vi "Create.vi"(6 "RH?":bool, 8 "Error In":errorcluster) -> (0 "error out":errorcluster)   [LabVIEW 2017]
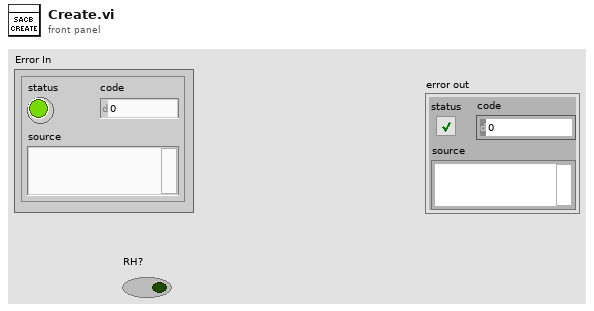
[diagram p1: front panel]
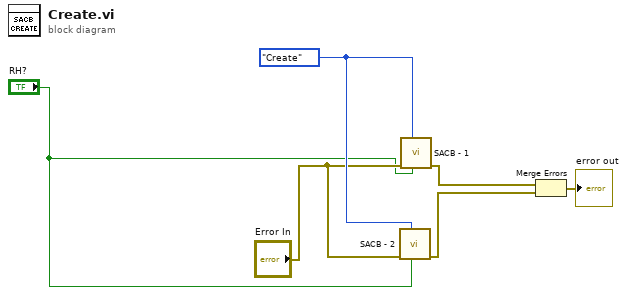
[diagram p0: block diagram]
diagram:
  w6 = enum16{"Create", "Read", "Close"}."Create" ("Command")
  n1 = call "SACB - 2.vi"("RH?"="RH?", "Command"=w6, "Error In"="Error In") -> ("Error Out"=w4:errorcluster)  [unwired: 7 in, 1 out]
  n2 = call "SACB - 1.vi"("RH?"="RH?", "Command"=w6, "Error In"="Error In") -> ("Error Out"=w5:errorcluster)  [unwired: 7 in, 1 out]
  n3 = Merge Errors(w5, w4) -> (→"error out":errorcluster)
